vi "automated room.vi"() -> ()   [LabVIEW 2026]
uses:
  <vilib>/numeric/Random Number (Range) U64.vi
  <vilib>/numeric/sub_Random U32.vi
panel:
  out "fan":bool
  out "switch":bool
  out "light psi":u64
  out "light psi":u64
  out "light  2":bool
  out "Boolean 2":bool
  out "light":bool
  out "Boolean":bool
  out "temp":u64
  out "switch":bool
  in  "stop":bool
  out "ac":bool
  in  "Enum":enum16{"ac", "light 2", "light 1", "fan"}(ring)
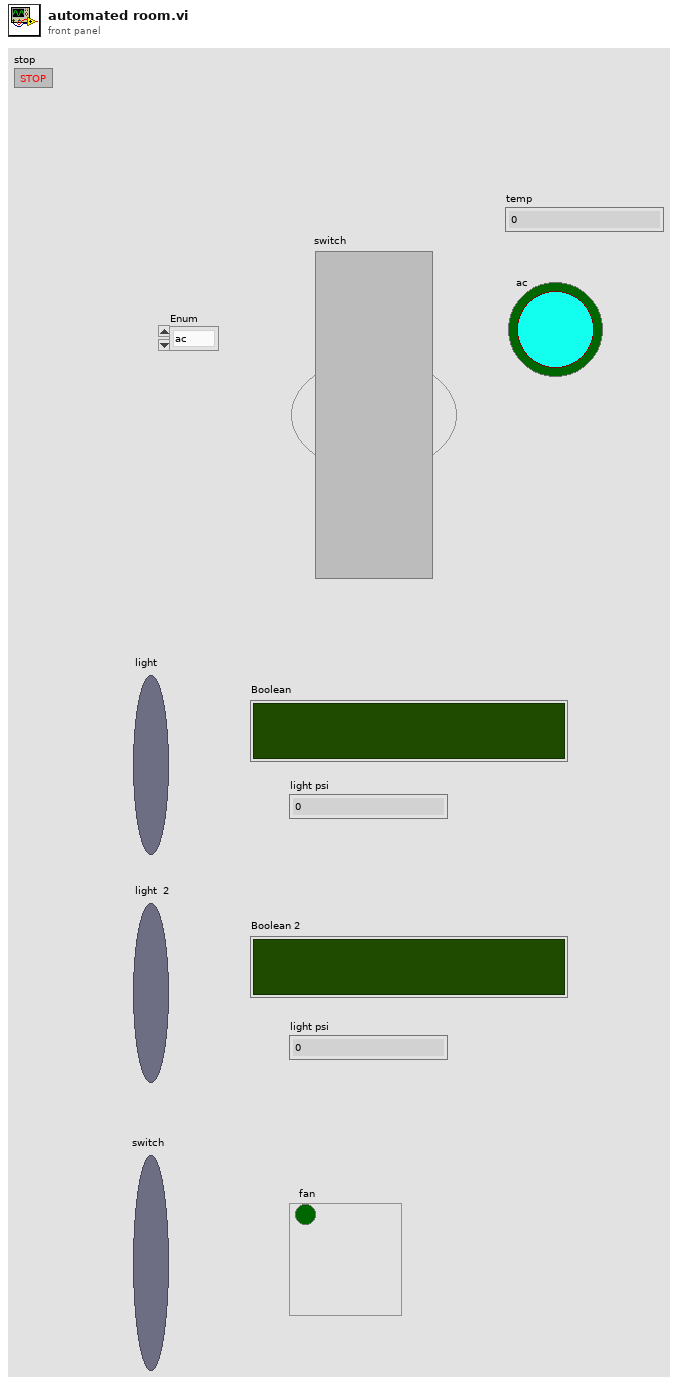
[diagram p1: front panel]
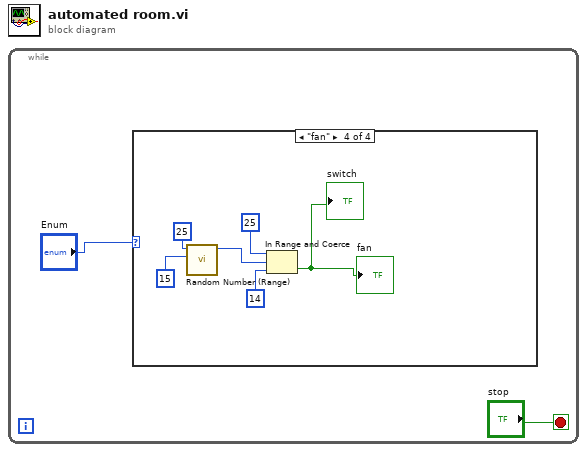
[diagram p0: block diagram]
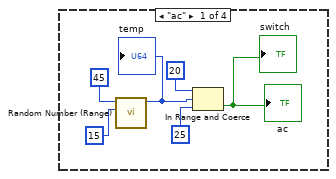
[diagram p2: hidden frame]
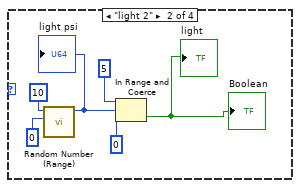
[diagram p3: hidden frame]
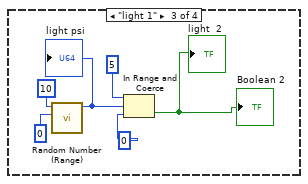
[diagram p4: hidden frame]
diagram:
  n1 = while {
    stop <- "stop" stop-if-true
    n2 = case shown="\"fan\"" "Enum" {
      frame "ac" {
        n3 = call-poly <vilib>:"Random Number (Range).vi"("lower bound (0)"=u64 15, "upper bound (100)"=u64 45) -> ("number"=w3:u64)  [unwired: 9 in]
        "temp" <- w3
        n4 = In Range and Coerce(upper limit=u64 20, x=w3, lower limit=u64 25) -> (In Range?=→"ac" →"switch":bool)  [unwired: 1 out]
      }
      frame "light 2" {
        n5 = call-poly <vilib>:"Random Number (Range).vi"("lower bound (0)"=u64 0, "upper bound (100)"=u64 10) -> ("number"=w9:u64)  [unwired: 9 in]
        "light psi" <- w9
        n6 = In Range and Coerce(upper limit=u64 5, x=w9, lower limit=u64 0) -> (In Range?=→"Boolean" →"light":bool)  [unwired: 1 out]
      }
      frame "light 1" {
        n7 = call-poly <vilib>:"Random Number (Range).vi"("lower bound (0)"=u64 0, "upper bound (100)"=u64 10) -> ("number"=w15:u64)  [unwired: 9 in]
        "light psi" <- w15
        n8 = In Range and Coerce(upper limit=u64 5, x=w15, lower limit=u64 0) -> (In Range?=→"Boolean 2" →"light  2":bool)  [unwired: 1 out]
      }
      frame "fan" {
        n9 = call-poly <vilib>:"Random Number (Range).vi"("lower bound (0)"=u64 15, "upper bound (100)"=u64 25) -> ("number"=w24:u64)  [unwired: 9 in]
        n10 = In Range and Coerce(upper limit=u64 25, x=w24, lower limit=u64 14) -> (In Range?=→"switch" →"fan":bool)  [unwired: 1 out]
      }
    }
  }
